vi "queue_message_New.vi"(2 "Array":dbl[](array[numeric]), 3 "message":string, 4 "queue_name":string) -> (0 "Queue_Successed":bool, 1 "queue_name_copy":string)   [LabVIEW 2018]
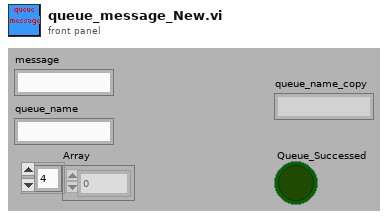
[diagram p1: front panel]
types:
  T1 = typedef "Queue RefNum" = refnum<k1>
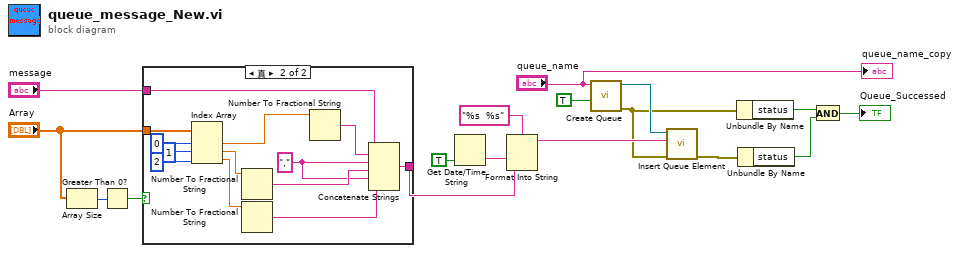
[diagram p0: block diagram]
diagram:
  n1 = Array Size(array="Array") -> (size(s)=w9:i32)
  n2 = Greater Than 0?(x=w9) -> (x > 0?=w7:bool)
  n3 = case shown="真" w7 {
    tunnel: [w18 w25] -> w11
    tunnel: "Array" -> [_ w20]
    tunnel: "message" -> [w18 w19]
    frame False {
    }
    frame True {
      w27 = "," ("string")
      n4 = Index Array(array=w20, index #1=0 ("index"), index #2=1 ("index"), index #3=2 ("index")) -> (element #1=w30:dbl, element #2=w22:dbl, element #3=w21:dbl)
      n5 = Number To Fractional String(number=w22) -> (F-format string=w28:string)  [unwired: 3 in]
      n6 = Number To Fractional String(number=w21) -> (F-format string=w26:string)  [unwired: 3 in]
      n7 = Number To Fractional String(number=w30) -> (F-format string=w31:string)  [unwired: 3 in]
      n8 = Concatenate Strings(w19, w31, w27, w28, w27, w26) -> (w25:string)
    }
  }
  n9 = Get Date/Time String(want seconds? (F)=TRUE) -> (time string=w15:string)  [unwired: 2 in, 1 out]
  n10 = Format Into String(format string="%s  %s", w15, w11) -> (resulting string=w16:string)  [unwired: 2 in, 1 out]
  n11 = call <vilib>:"Create Queue.vi"("return existing (F)"=TRUE ("return exisiting (F)"), "name (unnamed)"="queue_name") -> ("error out"=w6:errorcluster, "queue out"=w13:T1)  [unwired: 3 in, 1 out]
  n12 = call <vilib>:"Insert Queue Element.vi"("error in (no error)"=w6, "queue element"=w16, "queue"=w13) -> ("error out"=w5:errorcluster)  [unwired: 4 in, 2 out]
  n13 = Unbundle By Name(w6) -> ("status"=w4:bool)
  n14 = Unbundle By Name(w5) -> ("status"=w3:bool)
  n15 = And(x=w4, y=w3) -> (x .and. y?=→"Queue_Successed":bool)
  "queue_name_copy" <- "queue_name"
